vi "Write To Disk.vi"(8 "error in (no error)":errorcluster, 10 "Result In":string[][](array[string]), 11 "csv-formatter in":refnum<class "csv-formatter.lvclass">) -> (0 "error out":errorcluster, 3 "csv-formatter out":refnum<class "csv-formatter.lvclass">)   [LabVIEW 2015, in "csv-formatter.lvclass"]
uses:
  csv-formatter.lvclass
  csv-formatter.lvclass/csv-formatter.ctl
  <vilib>/Utility/file.llb/Write Delimited Spreadsheet (string).vi
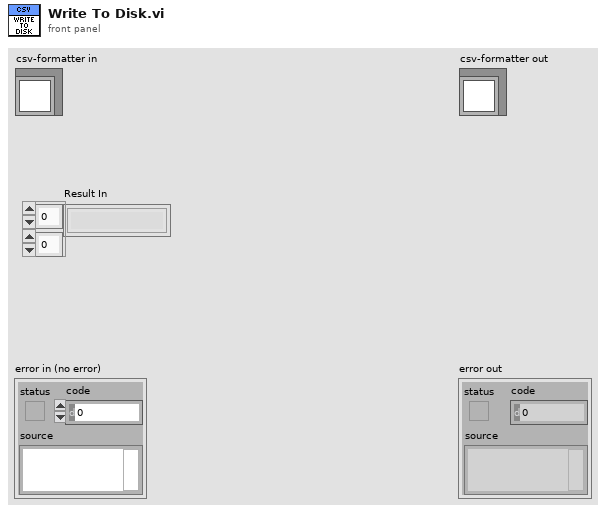
[diagram p1: front panel]
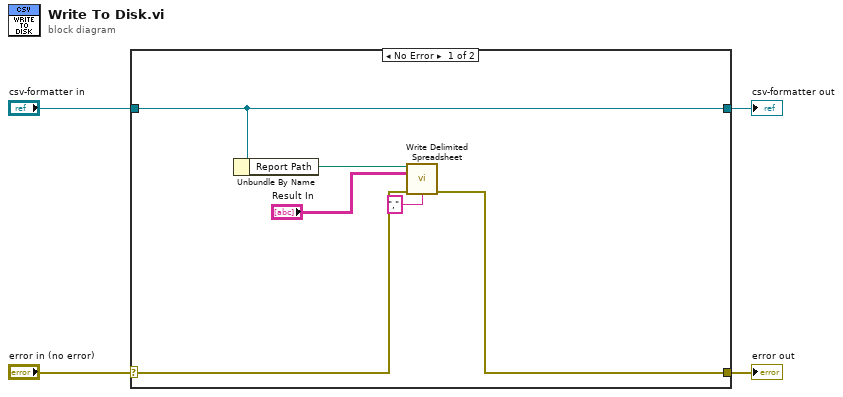
[diagram p0: block diagram]
diagram:
  n1 = case shown="No Error" "error in (no error)" {
    selector: "error in (no error)" -> [w8 w12]
    tunnel: [w7 w12] -> w3
    tunnel: [w10 w11] -> w1
    tunnel: "csv-formatter in" -> [w10 w11]
    frame No Error {
      n2 = Unbundle By Name(w10) -> ("Report Path"=w9:path)
      n3 = call-poly <vilib>:"Write Delimited Spreadsheet.vi"("file path (dialog if empty)"=w9, "2D data"="Result In", "error in (no error)"=w8, "delimiter (\\t)"="," ("delimiter (\\t)")) -> ("error out"=w7:errorcluster)  [unwired: 10 in, 1 out]
    }
    frame Error {
    }
  }
  "error out" <- w3
  "csv-formatter out" <- w1
